vi "DetermineGoNogoTrial.vi"(1 "Go Trial Probability":dbl, 2 "MaxSuccessiveTrials":i16=3, 3 "Mouse Performance":i16[][](array[numeric])) -> (0 "Go_Nogo":bool)   [LabVIEW 2013]
doc: "Outputs 0, 120 or 240"
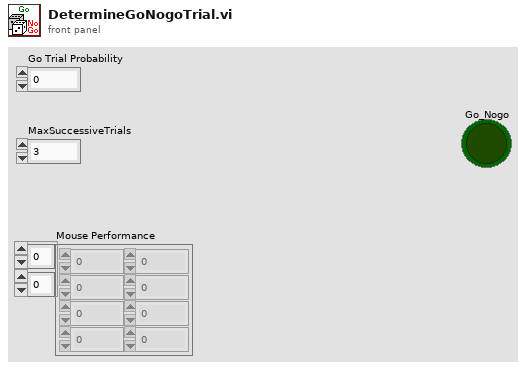
[diagram p1: front panel]
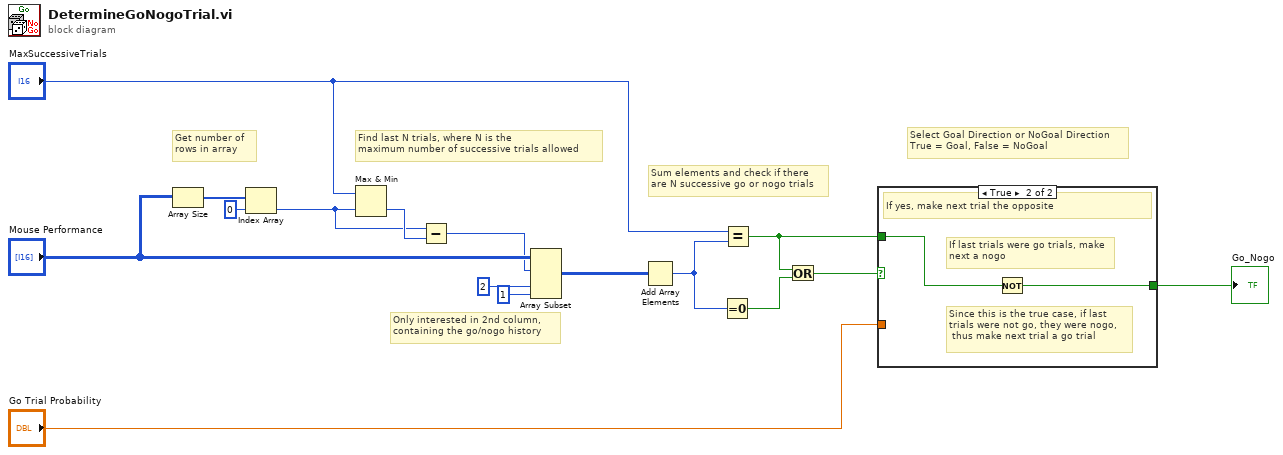
[diagram p0: block diagram]
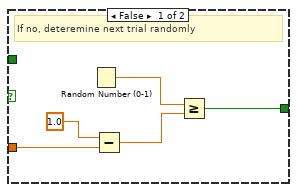
[diagram p2: hidden frame]
diagram:
  # "Sum elements and check if there \nare N successive go or nogo trials"
  # "Only interested in 2nd column, \ncontaining the go/nogo history"
  # "Find last N trials, where N is the \nmaximum number of successive trials allowed"
  # "Get number of \nrows in array"
  # "Select Goal Direction or NoGoal Direction\nTrue = Goal, False = NoGoal"
  n1 = Array Size(array="Mouse Performance") -> (size(s)=w16:i32[])
  n2 = Index Array(array=w16, index=0) -> (element=w9:i32)
  n3 = Max & Min(x="MaxSuccessiveTrials", y=w9) -> (min(x,y)=w14:i32)  [unwired: 1 out]
  n4 = Subtract(x=w9, y=w14) -> (x-y=w12:i32)
  n5 = Array Subset(array="Mouse Performance", index (row)=w12, index (col)=2 ("index"), length (col)=1 ("length")) -> (w7:i16[][])  [unwired: 1 in]
  n6 = Add Array Elements(numeric array=w7) -> (sum=w6:i16)
  n7 = Equal To 0?(x=w6) -> (x = 0?=w4:bool)
  n8 = Equal?(x="MaxSuccessiveTrials", y=w6) -> (x = y?=w1:bool)
  n9 = Or(x=w1, y=w4) -> (x .or. y?=w10:bool)
  n10 = case shown="True" w10 {
    tunnel: "Go Trial Probability" -> [w20 _]
    tunnel: [w17 w22] -> w2
    tunnel: w1 -> [_ w23]
    frame False {
      # "If no, deteremine next trial randomly"
      n11 = Random Number (0-1)() -> (number: 0 to 1=w19:dbl)
      n12 = Subtract(x=1.0, y=w20) -> (x-y=w18:dbl)
      n13 = Greater Or Equal?(x=w19, y=w18) -> (x >= y?=w17:bool)
    }
    frame True {
      # "Since this is the true case, if last\ntrials were not go, they were nogo,\n thus make next trial a go trial"
      # "If last trials were go trials, make\nnext a nogo"
      # "If yes, make next trial the opposite"
      n14 = Not(x=w23) -> (.not. x?=w22:bool)
    }
  }
  "Go_Nogo" <- w2
